vi "Configure Spectrum.vi"(6 "Jitter Line Resolution (0: jl256)":i32(ring) items=["jl256", "jl512", "jl1k", "jl2k", "jl4k", "jl8k"], 7 "Input Line Resolution (0: il512)":i32(ring) items=["il512", "il1k", "il2k", "il4k", "il8k", "il16k"], 8 "error in (no error)":errorcluster, 9 "Spectrum Window (0: BlkmanHarris)":i32(ring) items=["BlkmanHarris", "Hann", "Flattop", "EqRipple", "Uniform"], 10 "Calculate Spectrum (T: Enable)":bool=TRUE, 11 "VISA resource name":refnum<visa-resource-name>) -> (0 "error out":errorcluster, 3 "VISA resource name out":refnum<visa-resource-name>)   [LabVIEW 2014, in "Stanford Research SR1.lvlib"]
doc: "Configures the attributes for the Spectrum."
uses:
  Stanford Research SR1.lvlib
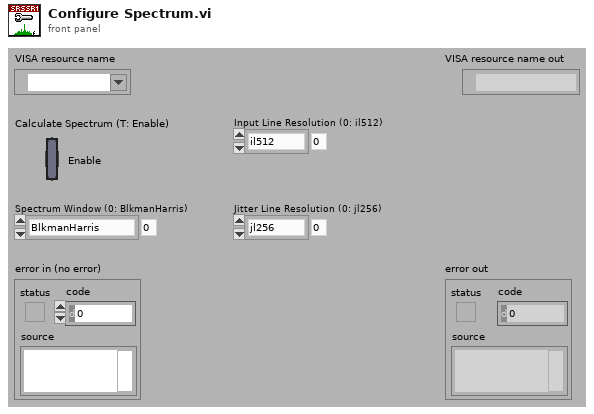
[diagram p1: front panel]
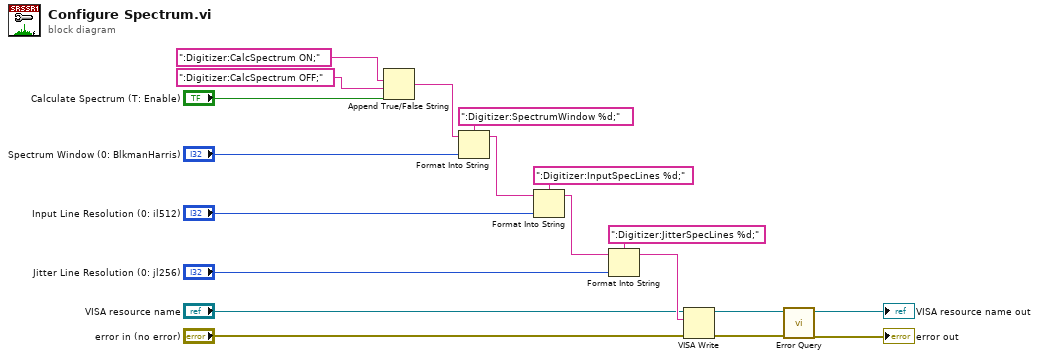
[diagram p0: block diagram]
diagram:
  n1 = Append True/False String(1:"Calculate Spectrum (T: Enable)", 2:":Digitizer:CalcSpectrum OFF;", 3:":Digitizer:CalcSpectrum ON;") -> (0:w16:string)  [unwired: 1 in]
  n2 = Format Into String(format string=":Digitizer:SpectrumWindow %d;", initial string=w16, "Spectrum Window (0: BlkmanHarris)") -> (resulting string=w13:string)  [unwired: 1 in, 1 out]
  n3 = Format Into String(format string=":Digitizer:InputSpecLines %d;", initial string=w13, "Input Line Resolution (0: il512)") -> (resulting string=w10:string)  [unwired: 1 in, 1 out]
  n4 = Format Into String(format string=":Digitizer:JitterSpecLines %d;", initial string=w10, "Jitter Line Resolution (0: jl256)") -> (resulting string=w7:string)  [unwired: 1 in, 1 out]
  n5 = VISA Write(VISA resource name="VISA resource name", write buffer=w7, error in (no error)="error in (no error)") -> (VISA resource name out=w4:refnum<visa-resource-name>, error out=w3:errorcluster)  [unwired: 1 out]
  n6 = call "Error Query.vi"("error in (no error)"=w3, "VISA resource name"=w4) -> ("error out"=→"error out":errorcluster, "VISA resource name out"=→"VISA resource name out":refnum<visa-resource-name>)  [unwired: 6 in, 2 out]
